vi "模拟量AD输入结果.vi"(8 "合格?":bool, 10 "第几个":i32) -> ()   [LabVIEW 2010]
uses:
  全局量/自动测试结果.vi
panel:
  # "从0开始"
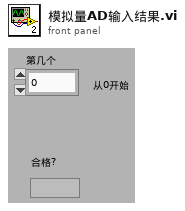
[diagram p1: front panel]
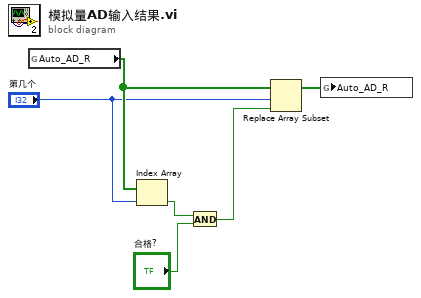
[diagram p0: block diagram]
diagram:
  n1 = global read "自动测试结果.vi" "Auto_AD_R"() -> (w4:bool[])
  n2 = Index Array(array=w4, index="第几个") -> (element=w6:bool)
  n3 = And(x=w6, y="合格?") -> (x .and. y?=w3:bool)
  n4 = Replace Array Subset(array=w4, new element=w3, index="第几个") -> (w2:bool[])
  n5 = global write "自动测试结果.vi" "Auto_AD_R"(w2) -> ()
